vi "CLD 10 Step Sequencer with CSV Solution.vi"() -> ()   [LabVIEW 2025]
doc: "CLD 10 Exercise\n\nUsing the state machine from CLD 9 and the FGV from CLD 6 exercise shortens the development time for this exercise."
uses:
  CLD 10 CSV file read eum.ctl
  CLD 10 CSV file data structure.ctl
  CLD 10 CSV file enum.ctl
panel:
  out "Current Step time":dbl
  out "Elapsed Time (s)":dbl format="%#.2g"
  out "Step 3":bool
  out "Step 2":bool
  out "Step 1":bool
  out "Time Has Elapsed":bool
  in  "Auto Reset":bool=TRUE
  in  "Reset Button":bool
  in  "Stop VI":bool
  out "error out":errorcluster
  in  "error in (no error)":errorcluster
  in  "Time Target (s)":dbl
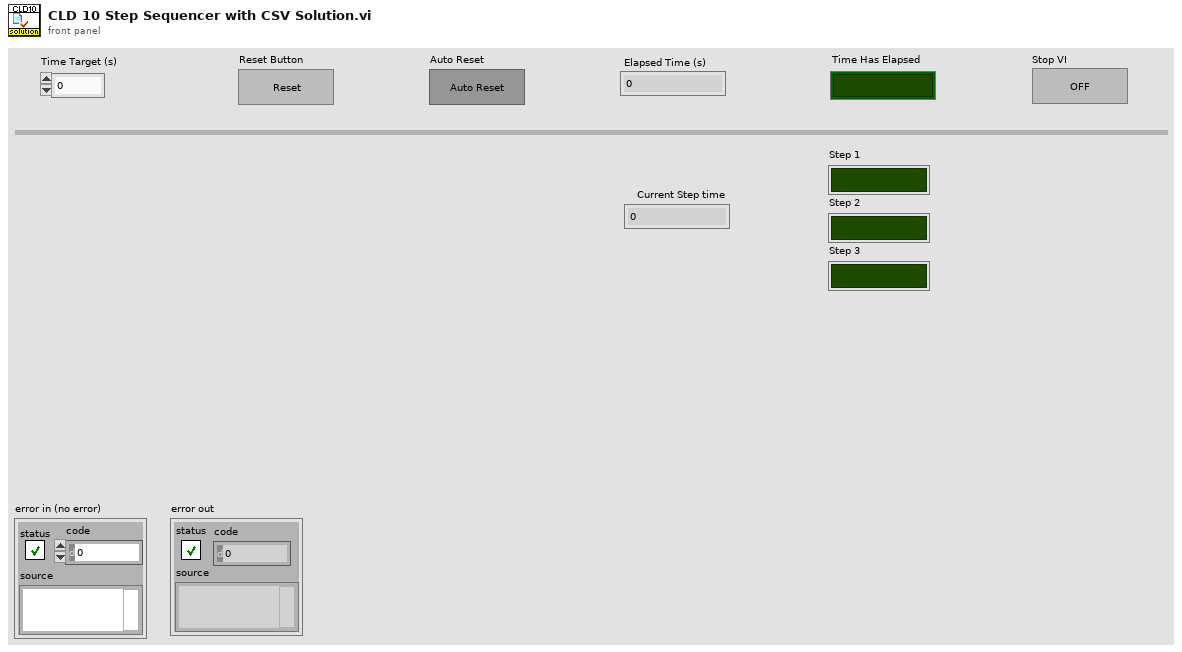
[diagram p1: front panel]
types:
  T1 = typedef "CLD 10 CSV file data structure.ctl" = cluster{"Step Time Target":i32, "Step 1":bool, "Step 2":bool, "Step 3":bool}
  T2 = typedef "CLD 10 CSV file read eum.ctl" = enum16{"Read CSV File", "Run Step One", "Run Step Two", "Run Step Three"}
  T3 = typedef "CLD 10 CSV file enum.ctl" = enum16{"Read CSV", "Write CSV"}
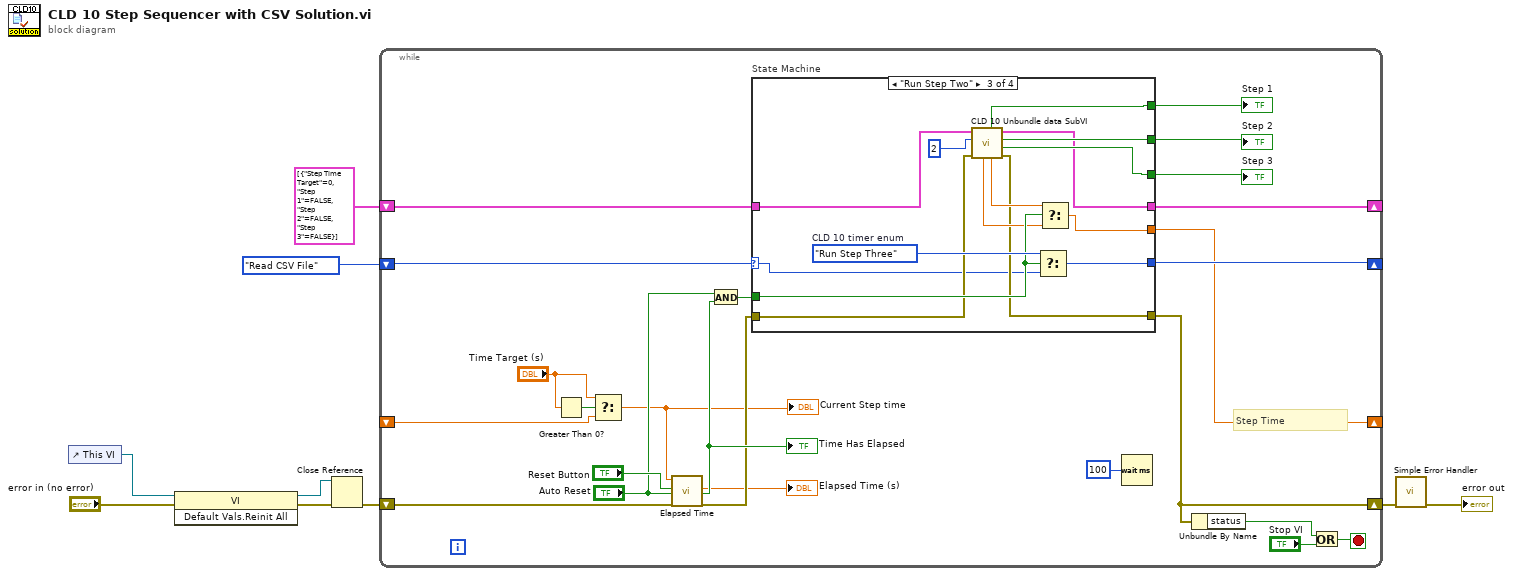
[diagram p0: block diagram]
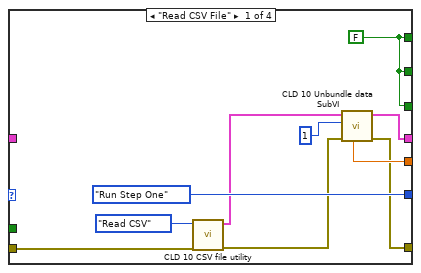
[diagram p2: hidden frame]
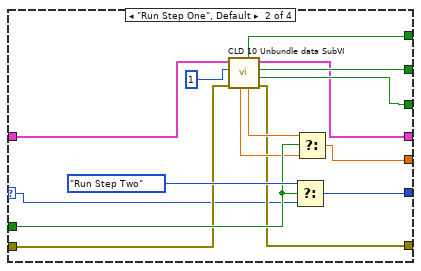
[diagram p3: hidden frame]
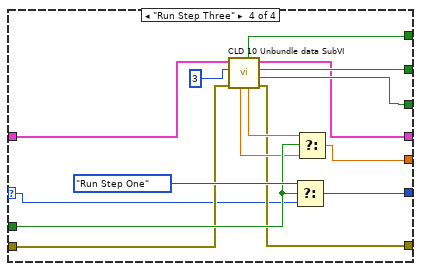
[diagram p4: hidden frame]
diagram:
  n1 = control-ref of="This VI"() -> (w6:refnum<vi>)
  n2 = invoke class="VI" method="Default Vals.Reinit All"(reference=w6, error in="error in (no error)") -> (reference out=w4:refnum<vi>, error out=w7:errorcluster)  [unwired: 1 in, 1 out]
  n3 = Close Reference(reference=w4, error in (no error)=w7) -> (error out=w5:errorcluster)
  n4 = while {
    shift-right: [w11] -> w8
    shift-left: w5 -> [w31]
    shift-right: [w29] -> _
    shift-left: CLD_10_CSV_file_read_eum."Read CSV File" ("Enum") -> [w28]
    shift-right: [w21] -> _
    shift-left: _ -> [w20]
    shift-right: [w15] -> _
    shift-left: T1[] [{"Step Time Target"=0, "Step 1"=FALSE, "Step 2"=FALSE, "Step 3"=FALSE}] ("[Data Out]") -> [w14]
    stop <- w17 stop-if-true
    # "Step Time"
    n5 = Greater Than 0?(x="Time Target (s)") -> (x > 0?=w23:bool)
    n6 = Select(t="Time Target (s)", s=w23, f=w20) -> (s? t:f=w12:dbl)
    "Current Step time" <- w12
    n7 = call "Elapsed Time"("Time Target (s)"=w12, "Reset"="Reset Button", "Auto Reset"="Auto Reset", "error in (no error)"=w31) -> ("Elapsed Time (s)"=→"Elapsed Time (s)":dbl, "Time has Elapsed"=w27:bool, "error out"=w13:errorcluster)  [unwired: 8 in, 5 out]
    "Time Has Elapsed" <- w27
    n8 = And(x="Auto Reset", y=w27) -> (x .and. y?=w19:bool)
    n9 = case "State Machine" shown="\"Run Step Two\"" w28 {
      selector: w28 -> [_ w46 w61 w76]
      tunnel: [CLD_10_CSV_file_read_eum."Run Step One" ("Enum") w57 w72 w87] -> w29
      tunnel: w19 -> [_ w56 w71 w86]
      tunnel: [w42 w45 w60 w75] -> w26
      tunnel: [w42 w50 w65 w80] -> w25
      tunnel: [w42 w49 w64 w79] -> w24
      tunnel: [w37 w55 w70 w85] -> w21
      tunnel: [w36 w44 w59 w74] -> w15
      tunnel: w14 -> [_ w54 w69 w84]
      tunnel: w13 -> [w40 w48 w63 w78]
      tunnel: [w34 w47 w62 w77] -> w11
      frame "Read CSV File" {
        w42 = FALSE
        n10 = call "CLD 10 CSV file utility.vi"("Error In"=w40, "CSV File Enum"=CLD_10_CSV_file_enum."Read CSV") -> ("Error Out"=w35:errorcluster, "[Data Out]"=w39:T1[])  [unwired: 8 in]
        n11 = call "CLD 10 Unbundle data SubVI.vi"("error in (no error)"=w35, "Current State Number"=1 ("State Number"), "[Data In]"=w39) -> ("error out"=w34:errorcluster, "[Data Out]"=w36:T1[], "Dwell Time"=w37:dbl)  [unwired: 2 in, 4 out]
      }
      frame "Run Step One", Default {
        n12 = call "CLD 10 Unbundle data SubVI.vi"("error in (no error)"=w48, "Current State Number"=1 ("State Number"), "[Data In]"=w54) -> ("error out"=w47:errorcluster, "State 3"=w49:bool, "State 2"=w50:bool, "[Data Out]"=w44:T1[], "Next Dwell Time"=w52:dbl, "State 1"=w45:bool, "Dwell Time"=w51:dbl)  [unwired: 2 in]
        n13 = Select(t=CLD_10_CSV_file_read_eum."Run Step Two" ("CLD 10 Timer Enum"), s=w56, f=w46) -> (s? t:f=w57:T2)
        n14 = Select(t=w52, s=w56, f=w51) -> (s? t:f=w55:dbl)
      }
      frame "Run Step Two" {
        w73 = CLD_10_CSV_file_read_eum."Run Step Three"  # CLD 10 timer enum
        n15 = call "CLD 10 Unbundle data SubVI.vi"("error in (no error)"=w63, "Current State Number"=2 ("State Number"), "[Data In]"=w69) -> ("error out"=w62:errorcluster, "State 3"=w64:bool, "State 2"=w65:bool, "[Data Out]"=w59:T1[], "Next Dwell Time"=w67:dbl, "State 1"=w60:bool, "Dwell Time"=w66:dbl)  [unwired: 2 in]
        n16 = Select(t=w73, s=w71, f=w61) -> (s? t:f=w72:T2)
        n17 = Select(t=w67, s=w71, f=w66) -> (s? t:f=w70:dbl)
      }
      frame "Run Step Three" {
        n18 = call "CLD 10 Unbundle data SubVI.vi"("error in (no error)"=w78, "Current State Number"=3 ("State Number"), "[Data In]"=w84) -> ("error out"=w77:errorcluster, "State 3"=w79:bool, "State 2"=w80:bool, "[Data Out]"=w74:T1[], "Next Dwell Time"=w82:dbl, "State 1"=w75:bool, "Dwell Time"=w81:dbl)  [unwired: 2 in]
        n19 = Select(t=CLD_10_CSV_file_read_eum."Run Step One" ("CLD 10 timer enum"), s=w86, f=w76) -> (s? t:f=w87:T2)
        n20 = Select(t=w82, s=w86, f=w81) -> (s? t:f=w85:dbl)
      }
    }
    "Step 1" <- w26
    "Step 2" <- w25
    "Step 3" <- w24
    n21 = Wait (ms)(milliseconds to wait=u32 100) -> ()  [unwired: 1 out]
    n22 = Unbundle By Name(w11) -> ("status"=w16:bool)
    n23 = Or(x=w16, y="Stop VI") -> (x .or. y?=w17:bool)
  }
  n24 = call <vilib>:"Simple Error Handler.vi"("error in (no error)"=w8) -> ("error out"=→"error out":errorcluster)  [unwired: 4 in, 4 out]
